vi "S2C_Shared_Proc_Initialize.vi"(8 "Error In":errorcluster, 11 "Q-Name":string) -> (0 "Error Out":errorcluster, 3 "Q-Ref":refnum<queue>)   [LabVIEW 2024]
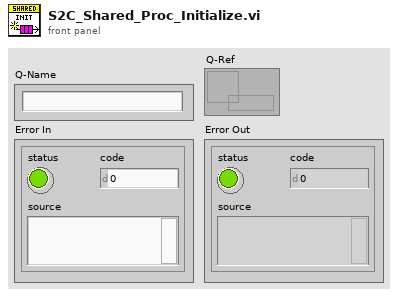
[diagram p1: front panel]
types:
  T1 = cluster{"Caller-Q":refnum<queue>, "Command":string, "Return":string, "Data":variant, "Timeout":dbl}
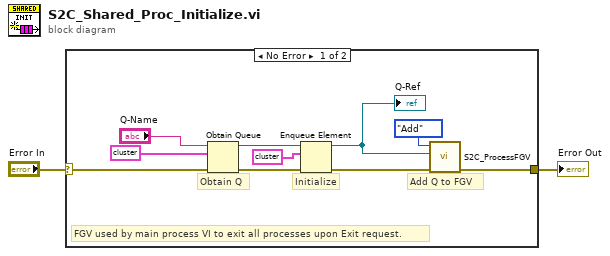
[diagram p0: block diagram]
diagram:
  n1 = case shown="No Error" "Error In" {
    selector: "Error In" -> [w10 w13]
    tunnel: [w5 w13] -> w1
    frame No Error {
      # "FGV used by main process VI to exit all processes upon Exit request."
      # "Add Q to FGV"
      # "Initialize"
      # "Obtain Q"
      n2 = Obtain Queue(name (unnamed)="Q-Name", element data type=T1 {"Caller-Q"=refnum, "Command"="", "Return"="", "Data"=variant, "Timeout"=0.0} ("Command Cluster"), error in (no error)=w10) -> (queue out=w11:refnum<queue>, error out=w12:errorcluster)  [unwired: 2 in, 1 out]
      n3 = Enqueue Element(queue=w11, element=T1 {"Caller-Q"=refnum, "Command"="^Init", "Return"="", "Data"=variant, "Timeout"=0.0} ("Command Cluster"), error in (no error)=w12) -> (queue out=w3:refnum<queue>, error out=w6:errorcluster)  [unwired: 1 in, 1 out]
      "Q-Ref" <- w3
      n4 = call "S2C_ProcessFGV.vi"("Error In"=w6, "Q-Ref"=w3, "Action"=enum16{"Init", "Add", "Get"}."Add") -> ("Error Out"=w5:errorcluster)  [unwired: 7 in, 1 out]
    }
    frame Error {
    }
  }
  "Error Out" <- w1
